vi "Write Display_Ref.vi"(8 "error in (no error)":errorcluster, 10 "Display_Ref":refnum<vi>, 11 "DAQ970 in":refnum<class "DAQ970.lvclass">) -> (0 "error out":errorcluster, 3 "DAQ970 out":refnum<class "DAQ970.lvclass">)   [LabVIEW 2019, in "DAQ970.lvlib" / "DAQ970.lvclass"]
uses:
  Library/DAQ970.lvclass
  Library/DAQ970.lvclass/DAQ970.ctl
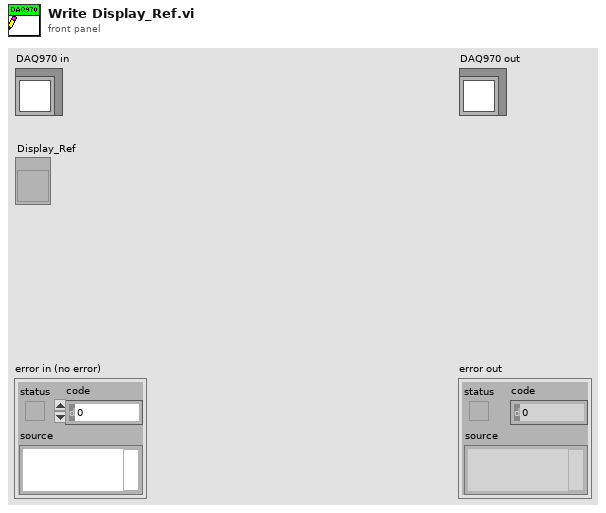
[diagram p1: front panel]
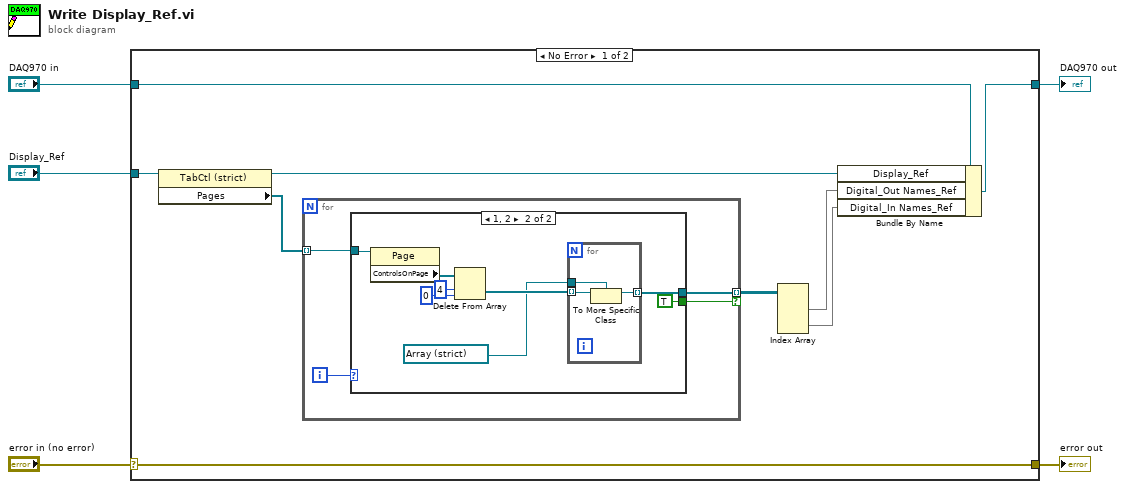
[diagram p0: block diagram]
diagram:
  n1 = case shown="No Error" "error in (no error)" {
    selector: "error in (no error)" -> [w14 w30]
    tunnel: [w14 w30] -> w4
    tunnel: [w12 w31] -> w2
    tunnel: "DAQ970 in" -> [w13 w31]
    tunnel: "Display_Ref" -> [w11 _]
    frame No Error {
      n2 = property class="TabCtl (strict)"(reference=w11) -> (reference out=w10:refnum<vi>, "Pages"=w9:refnum<vi>[])  [unwired: 1 in, 1 out]
      n3 = for {
        tunnel: w9 -> [w17] mode=indexing
        tunnel: [w16] -> w8 mode=indexing if=w15
        i -> [w18]
        n4 = case shown="1, 2" w18 {
          tunnel: w17 -> [_ w26]
          tunnel: [_ TRUE] -> w15
          tunnel: [_ w20] -> w16
          frame 0, Default {
          }
          frame 1, 2 {
            n5 = property class="Page"(reference=w26) -> ("ControlsOnPage"=w25:refnum<vi>[])  [unwired: 1 in, 2 out]
            n6 = Delete From Array(array=w25, length=4, index=0) -> (deleted portion=w21:refnum<vi>[])  [unwired: 1 out]
            n7 = for {
              tunnel: w21 -> [w29] mode=indexing
              tunnel: [w27] -> w20 mode=indexing
              tunnel: refnum<vi> refnum ("Digital_In Names") -> [w28]
              n8 = To More Specific Class(target class=w28, reference=w29) -> (specific class reference=w27:refnum<vi>)  [unwired: 1 in, 1 out]
            }
          }
        }
      }
      n9 = Index Array(array=w8) -> (element #1=w7:refnum<vi>[], element #2=w6:refnum<vi>[])  [unwired: 4 in]
      n10 = Bundle By Name(cluster=w13, "Display_Ref"=w10, "Digital_Out Names_Ref"=w7, "Digital_In Names_Ref"=w6) -> (w12:refnum<class "DAQ970.lvclass">)
    }
    frame Error {
    }
  }
  "error out" <- w4
  "DAQ970 out" <- w2
